vi "Convert Device Units to Acceleration Units.vi"(9 "Microstep Size (0)":dbl, 10 "Units (0: device acceleration units)":u16(ring) items=["device acceleration units", "microsteps per second squared", "microns per second squared", "millimeters per second squared", "inches per second squared", "degrees per second squared"], 11 "Device Acceleration (0)":i32) -> (3 "Acceleration":dbl)   [LabVIEW 2018, in "Zaber A Series.lvlib"]
doc: "Helper to convert device-specific units of acceleration to standard units.\n\nSelect a unit and enter an a device's acceleration quantity. The output will be the acceleration converted to the selected unit.\n\nIf you select a unit other than device units or microsteps per second squared, you must also provide the Microstep Size conversion factor from microsteps to micrometers, which can be found in your device manual.\n\nThis VI is deprecated in order to make the list of units consistent with speed and position VIs. Please use \"Convert Device Units to Acceleration\" instead."
uses:
  Zaber A Series.lvlib
panel:
  # "DEPRECATED\n \n This VI is deprecated in order to make the unit list consistent with\n other VIs.  Please use the new \"Convert Device Units to\n Acceleration\" VI instead."
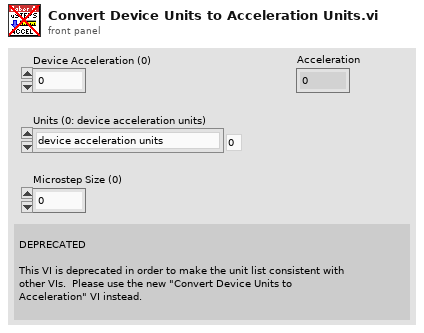
[diagram p1: front panel]
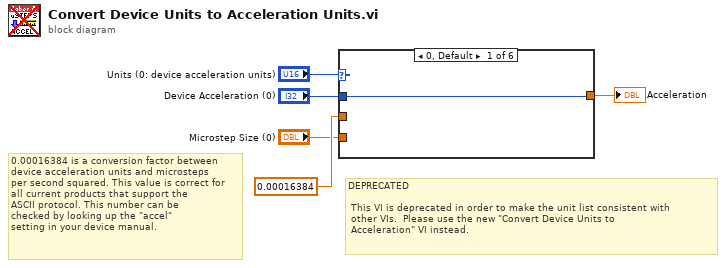
[diagram p0: block diagram]
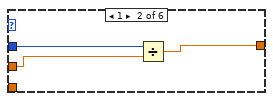
[diagram p2: hidden frame]
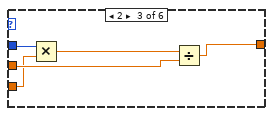
[diagram p3: hidden frame]
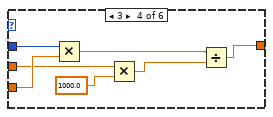
[diagram p4: hidden frame]
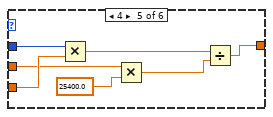
[diagram p5: hidden frame]
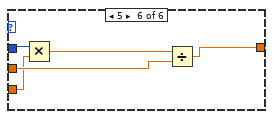
[diagram p6: hidden frame]
diagram:
  # "DEPRECATED\n \n This VI is deprecated in order to make the unit list consistent with\n other VIs.  Please use the new \"Convert Device Units to\n Acceleration\" VI instead."
  # "0.00016384 is a conversion factor between \ndevice acceleration units and microsteps \nper second squared. This value is correct for\nall current products that support the\nASCII protocol. This number can be \nchecked by looking up the \"accel\"\nsetting in your device manual."
  n1 = case shown="0, Default" "Units (0: device acceleration units)" {
    tunnel: 0.00016384 ("Acceleration Constant (0.00016384)") -> [_ w8 w13 w16 w23 w32]
    tunnel: "Microstep Size (0)" -> [_ _ w11 w17 w26 w29]
    tunnel: [w6 w7 w10 w15 w28 w31] -> w1
    tunnel: "Device Acceleration (0)" -> [w6 w9 w12 w18 w27 w30]
    frame 0, Default {
    }
    frame 1 {
      n2 = Divide(x=w9, y=w8) -> (x/y=w7:dbl)
    }
    frame 2 {
      n3 = Multiply(x=w12, y=w11) -> (x*y=w14:dbl)
      n4 = Divide(x=w14, y=w13) -> (x/y=w10:dbl)
    }
    frame 3 {
      n5 = Multiply(x=w18, y=w17) -> (x*y=w20:dbl)
      n6 = Multiply(x=w16, y=1000.0) -> (x*y=w21:dbl)
      n7 = Divide(x=w20, y=w21) -> (x/y=w15:dbl)
    }
    frame 4 {
      n8 = Multiply(x=w27, y=w26) -> (x*y=w25:dbl)
      n9 = Multiply(x=w23, y=25400.0) -> (x*y=w22:dbl)
      n10 = Divide(x=w25, y=w22) -> (x/y=w28:dbl)
    }
    frame 5 {
      n11 = Multiply(x=w30, y=w29) -> (x*y=w33:dbl)
      n12 = Divide(x=w33, y=w32) -> (x/y=w31:dbl)
    }
  }
  "Acceleration" <- w1
